vi "AUTO_STATE_QUEUE.vi"(7 "QUEUE ST":T2=enum."CLOSE Q", 8 "error in":errorcluster, 11 "AUTO ST":T1[](array[typedef])=[enum."Int"]) -> (0 "error OUT":errorcluster, 3 "Enum":T1)   [LabVIEW 2017]
uses:
  Controls/AUTO_STATE_QUEUE.ctl
  Controls/Ass. Loop Control.ctl
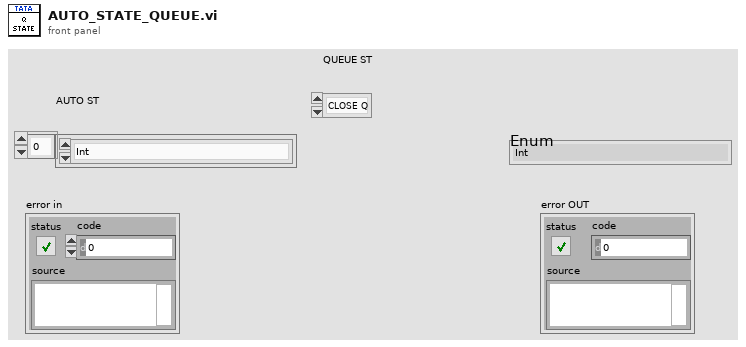
[diagram p1: front panel]
types:
  T1 = typedef "Ass. Loop Control.ctl" = enum16{"Int", "Int2", "Cluster_update", "Wait", "BOX_at_Filling_Station", "Scan_LH_Code", "Scan_RH_Code", "STATION1_Start Cycle", "STATION_1_SCAN", "STATION1_barcode CHECK", "STATION1_SaveDATA_sql", "STATION1_Cycle End", "STATION1_Cycle_Cancle", "STATION2_SCAN", "STATION2_SaveDATA_sql", "Stop", "Error Handler"}
  T2 = typedef "AUTO_STATE_QUEUE.ctl" = enum16{"CREATE Q", "EN Q", "DE Q", "CLOSE Q"}
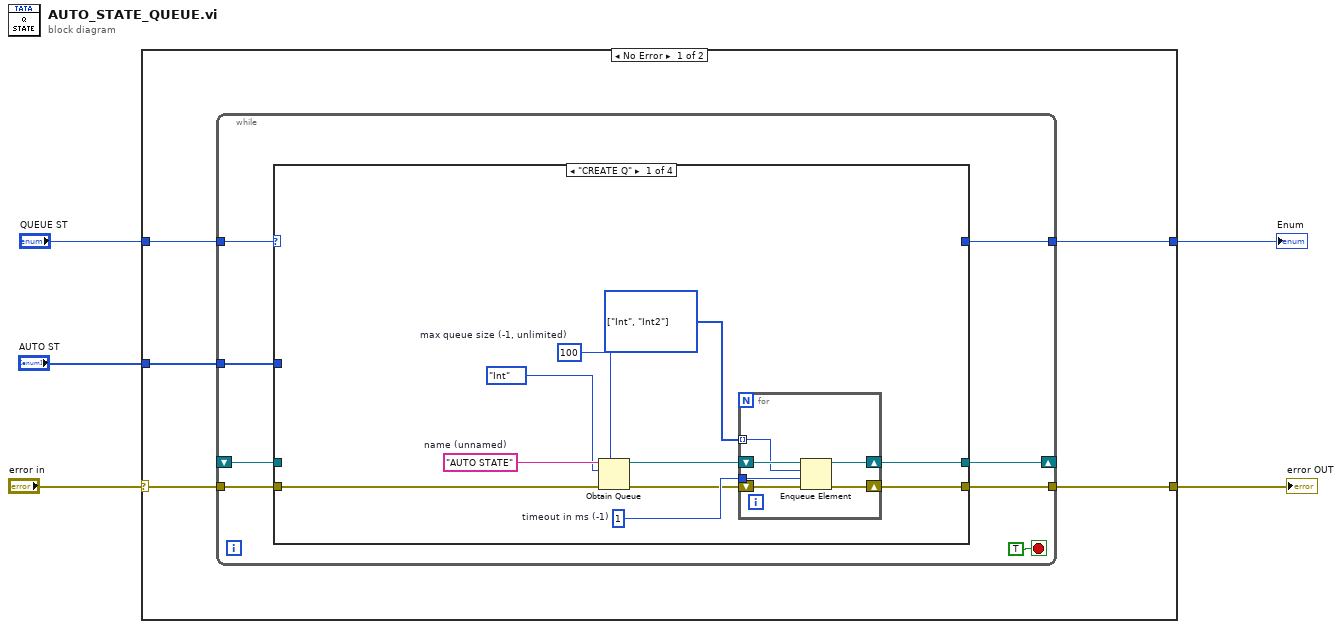
[diagram p0: block diagram]
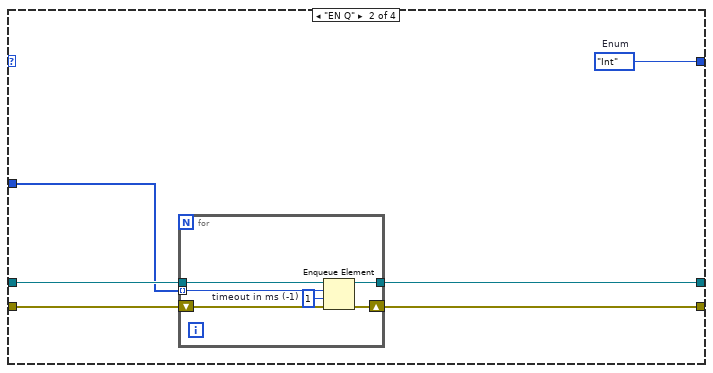
[diagram p2: hidden frame]
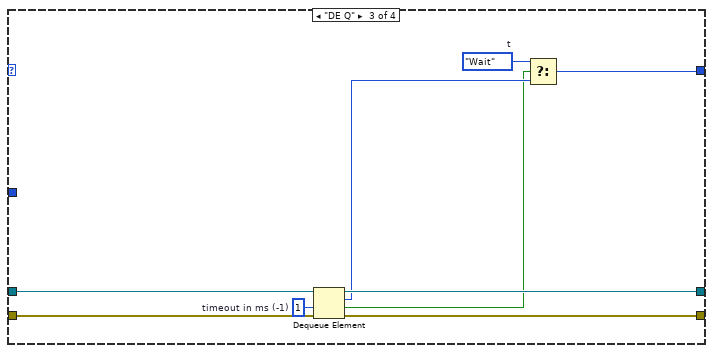
[diagram p3: hidden frame]
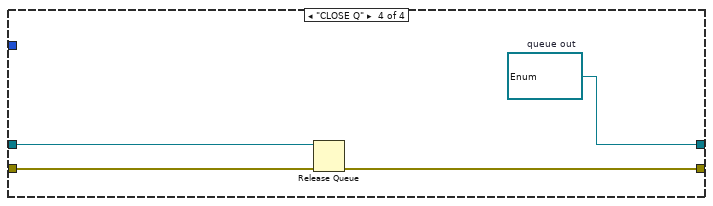
[diagram p4: hidden frame]
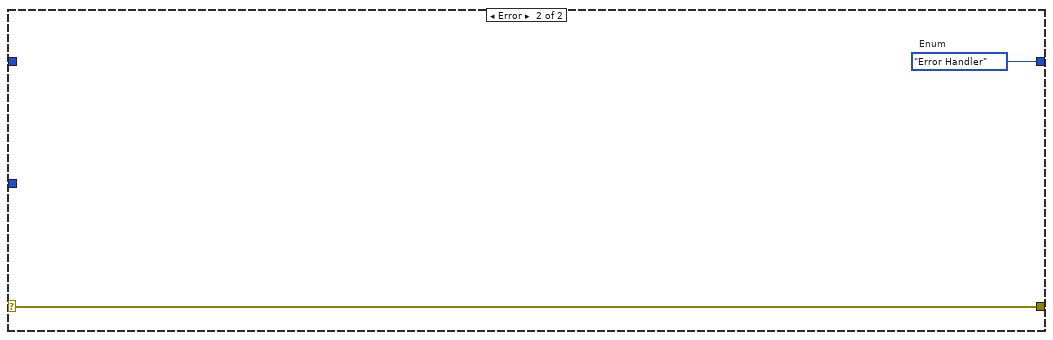
[diagram p5: hidden frame]
diagram:
  n1 = case shown="No Error" "error in" {
    selector: "error in" -> [w10 w61]
    tunnel: [w9 w61] -> w4
    tunnel: [w8 w60] -> w1
    tunnel: "QUEUE ST" -> [w7 _]
    tunnel: "AUTO ST" -> [w6 _]
    frame No Error {
      n2 = while {
        tunnel: w10 -> [w18]
        tunnel: [w16] -> w9
        tunnel: [w11] -> w8
        tunnel: w7 -> [w15]
        shift-right: [w14] -> _
        shift-left: _ -> [w13]
        tunnel: w6 -> [w12]
        stop <- TRUE stop-if-true
        n3 = case shown="\"CREATE Q\"" w15 {
          tunnel: w18 -> [w28 w40 w55 w59]
          tunnel: [w20 w39 w54 w58] -> w16
          tunnel: [w22 w37 w52 w56] -> w14
          tunnel: w13 -> [_ w38 w53 w57]
          tunnel: w12 -> [_ w36 _ _]
          tunnel: [_ w35 w49 _] -> w11
          frame "CREATE Q" {
            w19 = T1[] [enum."Int", enum."Int2"] items=["Int", "Int2", "Cluster_update", "Wait", "BOX_at_Filling_Station", "Scan_LH_Code", "Scan_RH_Code", "STATION1_Start Cycle", "STATION_1_SCAN", "STATION1_barcode CHECK", "STATION1_SaveDATA_sql", "STATION1_Cycle End", "STATION1_Cycle_Cancle", "STATION2_SCAN", "STATION2_SaveDATA_sql", "Stop", "Error Handler"] ("Array")
            w24 = 1  # timeout in ms (-1)
            w26 = 100  # max queue size (-1, unlimited)
            w27 = "AUTO STATE"  # name (unnamed)
            n4 = Obtain Queue(max queue size (-1, unlimited)=w26, name (unnamed)=w27, element data type=Ass._Loop_Control."Int" ("Enum"), error in (no error)=w28) -> (queue out=w23:refnum<queue>, error out=w21:errorcluster)  [unwired: 1 in, 1 out]
            n5 = for {
              tunnel: w24 -> [w34]
              tunnel: w19 -> [w29] mode=indexing
              shift-right: [w32] -> w22
              shift-left: w23 -> [w33]
              shift-right: [w30] -> w20
              shift-left: w21 -> [w31]
              n6 = Enqueue Element(queue=w33, element=w29, timeout in ms (-1)=w34, error in (no error)=w31) -> (queue out=w32:refnum<queue>, error out=w30:errorcluster)  [unwired: 1 out]
            }
          }
          frame "EN Q" {
            w35 = Ass._Loop_Control."Int"  # Enum
            n7 = for {
              tunnel: w38 -> [w44]
              tunnel: [w43] -> w37
              tunnel: w36 -> [w42] mode=indexing
              shift-right: [w45] -> w39
              shift-left: w40 -> [w46]
              w41 = 1  # timeout in ms (-1)
              n8 = Enqueue Element(queue=w44, element=w42, timeout in ms (-1)=w41, error in (no error)=w46) -> (queue out=w43:refnum<queue>, error out=w45:errorcluster)  [unwired: 1 out]
            }
          }
          frame "DE Q" {
            w47 = Ass._Loop_Control."Wait"  # t
            w51 = 1  # timeout in ms (-1)
            n9 = Dequeue Element(queue=w53, timeout in ms (-1)=w51, error in (no error)=w55) -> (queue out=w52:refnum<queue>, element=w50:T1, timed out?=w48:bool, error out=w54:errorcluster)
            n10 = Select(t=w47, s=w48, f=w50) -> (s? t:f=w49:T1)
          }
          frame "CLOSE Q" {
            w56 = refnum<queue> refnum items=["Int", "Int2", "Cluster_update", "Wait", "BOX_at_Filling_Station", "Scan_LH_Code", "Scan_RH_Code", "STATION1_Start Cycle", "STATION_1_SCAN", "STATION1_barcode CHECK", "STATION1_SaveDATA_sql", "STATION1_Cycle End", "STATION1_Cycle_Cancle", "STATION2_SCAN", "STATION2_SaveDATA_sql", "Stop", "Error Handler"]  # queue out
            n11 = Release Queue(queue=w57, error in (no error)=w59) -> (error out=w58:errorcluster)  [unwired: 1 in, 2 out]
          }
        }
      }
    }
    frame Error {
      w60 = Ass._Loop_Control."Error Handler"  # Enum
    }
  }
  "error OUT" <- w4
  "Enum" <- w1
